vi "Real Inverse Matrix (Triangular).vi"(2 "matrix type":enum32{"lower triangular", "upper triangular"}(ring), 3 "A":T1) -> (0 "error":i32, 1 "Inverse Matrix":T1)   [LabVIEW 2017, in "NI_AALBase.lvlib"]
uses:
  NI_AALBase.lvlib
  RealMatrix.ctl
  <resource>/lvanlys.dll
  NI_Matrix.lvlib
panel:
  # "Real Inverse Matrix (Triangular)"
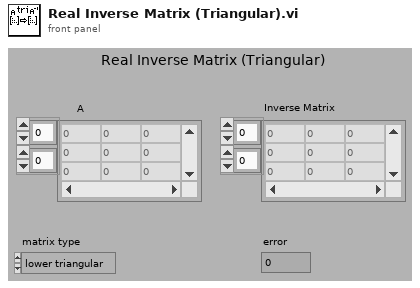
[diagram p1: front panel]
types:
  T1 = typedef "NI_Matrix.lvlib/RealMatrix.ctl" = dbl[][]
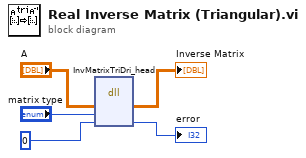
[diagram p0: block diagram]
diagram:
  n1 = dll-call lib="C:/Program Files (x86)/National Instruments/LabVIEW 2017/resource/lvanlys.*" fn="InvMatrixTriDri_head"("A"="A", "mtype"="matrix type", 0) -> ("A"=→"Inverse Matrix":T1, →"error":i32)  [unwired: 5 in, 2 out]
